vi "OneMacro_analog.vi"(3 "Task cluster in":T2={"Inbits"="Inbits", "Outbits"="Outbits", "Error Array"=[{"status"=FALSE, "code"=0, "source"=""}, {"status"=FALSE, "code"=0, "source"=""}, {"status"=FALSE, "code"=0, "source"=""}, {"status"=FALSE, "code"=0, "source"=""}, {"status"=FALSE, "code"=0, "source"=""}], "AO Array"=["AO 00-07", "AO 08-15", "AO 16-23"]}, 4 "RAW cmds 2D":i16[][](array[numeric])=[[5000, 0, 7, 5, 0, 3, -4, 5, 0, 0, 7, 5, 0, 3, -4, 5], [-4, -1, -5, 0, 0, 0, 0, 0, -4, -1, -5, 0, 0, 0, 0, 0], [0, 0, 0, 0, 0, 0, 0, 0, 0, 0, 0, 0, 0, 0, 0, 0]], 5 "Duration (s)":dbl=0.001) -> (0 "Task cluster out":T2={"Inbits"="Inbits", "Outbits"="Outbits", "Error Array"=[{"status"=FALSE, "code"=0, "source"=""}, {"status"=FALSE, "code"=0, "source"=""}, {"status"=FALSE, "code"=0, "source"=""}, {"status"=FALSE, "code"=0, "source"=""}, {"status"=FALSE, "code"=0, "source"=""}], "AO Array"=["AO 00-07", "AO 08-15", "AO 16-23"]})   [LabVIEW 2018]
uses:
  <vilib>/DAQmx/write.llb/DAQmx Write (Raw 1D I16).vi
  Tasks_RT.ctl
panel:
  in  "subvi?":bool
  in  "Single Instruction":T1={"Duration (s)"=0.01, "Instruction Description"="Set U11 to 50 V, set output bit 1 to high", "Input Bits"=[FALSE, FALSE, FALSE, FALSE, FALSE, FALSE, FALSE, FALSE, FALSE, FALSE, FALSE, FALSE, FALSE, FALSE, FALSE, FALSE], "Output Bits"=[TRUE, FALSE, FALSE, FALSE, FALSE, FALSE, FALSE, FALSE, FALSE, FALSE, FALSE, FALSE, FALSE, FALSE, FALSE, FALSE, FALSE, FALSE, FALSE, FALSE, FALSE, FALSE, FALSE, FALSE, FALSE, FALSE, FALSE, FALSE, FALSE, FALSE, FALSE, FALSE, FALSE, FALSE, FALSE, FALSE, FALSE, FALSE], "Excitations"=[-1.301715176715177, -0.0, 0.002243270189431705, 0.0014977533699450823, -0.0, 0.000996512207274539, -0.001245640259093174, 0.0014814814814814814, -0.0012431626056688216, -0.00024900398406374507, -0.0014903129657228018, -0.0, -0.0, -0.0, -0.0, -0.0, -0.0, -0.0, -0.0, -0.0, -0.0, -0.0, 0.0, 0.0], "Steps"=1, "Changes"=[FALSE, TRUE, TRUE]}
  # "Tasks and errors"
  # "Tasks and errors"
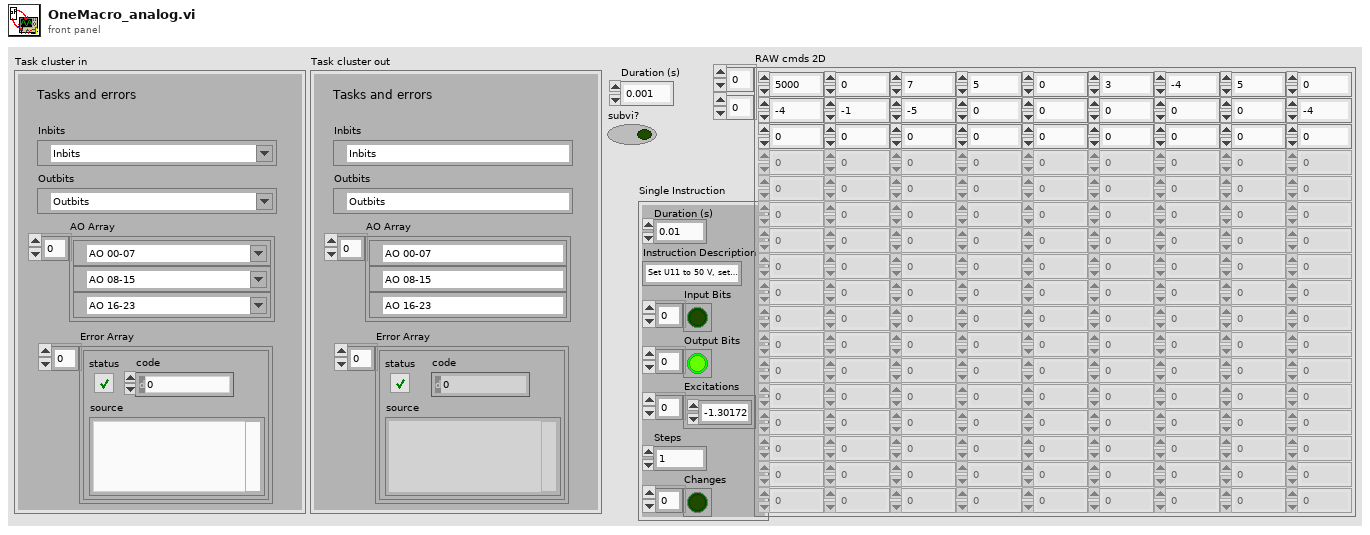
[diagram p1: front panel]
types:
  T1 = cluster{"Duration (s)":dbl, "Instruction Description":string, "Input Bits":bool[], "Output Bits":bool[], "Excitations":dbl[], "Steps":i32, "Changes":bool[]}
  T2 = typedef "Tasks.ctl" = cluster{"Inbits":refnum<k21>, "Outbits":refnum<k21>, "Error Array":errorcluster[], "AO Array":refnum<k21>[]}
  T3 = typedef "Tasks_RT.ctl" = cluster{"Outbits":refnum<k21>, "Error Array":errorcluster[], "Counter":refnum<k21>, "Slow AO":refnum<k21>, "Fast AO":refnum<k21>[], "Trigger":refnum<k21>}
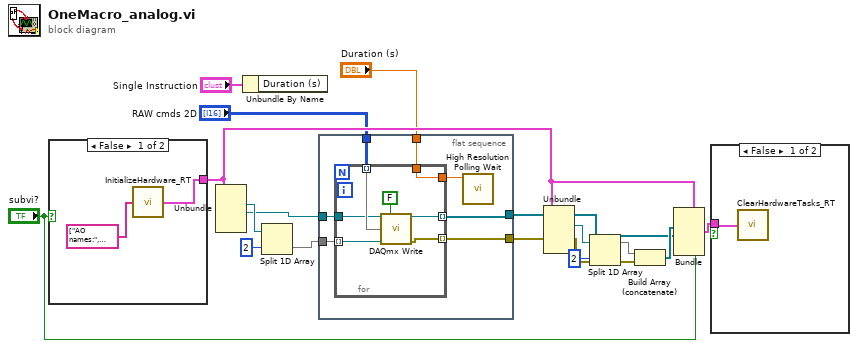
[diagram p0: block diagram]
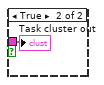
[diagram p2: hidden frame]
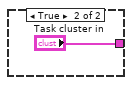
[diagram p3: hidden frame]
diagram:
  n1 = case shown="False" "subvi?" {
    tunnel: [w18 "Task cluster in"] -> w15
    frame False {
      n2 = call "InitializeHardware_RT.vi"("PXI card names"=string[] ["AO names:", "6733", "DIO name:", "6602"]) -> ("Task cluster"=w18:T3)
    }
    frame True {
    }
  }
  n3 = Unbundle(w15) -> ("Counter"=w13:refnum<k21>, "Slow AO"=w10:refnum<k21>)  [unwired: 4 out]
  n4 = Unbundle By Name("Single Instruction") -> ()  [unwired: 1 out]
  n5 = Split 1D Array(array=w13, index=2) -> (second subarray=w11:refnum<k21>[])  [unwired: 1 out]
  n6 = flat-sequence {
    tunnel: w11 -> [w26]
    tunnel: w10 -> [w25]
    tunnel: "RAW cmds 2D" -> [w24]
    tunnel: [w23] -> w4
    tunnel: [w22] -> w3
    tunnel: "Duration (s)" -> [w20]
    frame #0 {
      n7 = for {
        tunnel: w26 -> [w28] mode=indexing
        tunnel: w25 -> [w29]
        tunnel: [w33] -> w23 mode=indexing
        tunnel: [w32] -> w22 mode=indexing
        tunnel: w24 -> [w31] mode=indexing
        tunnel: [w30] -> w21
        tunnel: w20 -> [w30]
        n8 = call-poly <vilib>:"DAQmx Write.vi"("task/channels in"=w29, "auto start"=FALSE, "data"=w31, "error in"=w28) -> ("task out"=w33:refnum<k21>, "error out"=w32:errorcluster)  [unwired: 9 in, 1 out]
      }
      n9 = call <vilib>:"High Resolution Polling Wait.vi"("seconds to wait"=w21) -> ()  [unwired: 10 in, 1 out]
    }
  }
  n10 = Unbundle(w15) -> ("Counter"=w8:refnum<k21>)  [unwired: 5 out]
  n11 = Split 1D Array(array=w8, index=2) -> (first subarray=w7:refnum<k21>[])  [unwired: 1 out]
  n12 = Build Array (concatenate)(w7, w3) -> (w6:refnum<k21>[])
  n13 = Bundle(cluster=w15, "Counter"=w6, "Slow AO"=w4) -> (w14:T3)  [unwired: 4 in]
  n14 = case shown="False" "subvi?" {
    tunnel: w14 -> [w34 w35]
    frame False {
      n15 = call "ClearHardwareTasks_RT.vi"("Task cluster"=w34) -> ()  [unwired: 1 in]
    }
    frame True {
      "Task cluster out" <- w35
    }
  }
